vi "Save Results Time Steps.vi"() -> (5 "Plug in titles":string[](array[string]), 7 "Plug in values":string[](array[string]))   [LabVIEW 2020]
uses:
  <vilib>/Analysis/baseanly.llb/Mean (DBL).vi
  Globals/Meas_global.vi
  Globals/Dynamic_call_global.ph.vi
  <vilib>/Analysis/NI_AALBase.lvlib
  Controls/Post_Process.ctl
  Controls/Setup.ctl
panel:
  out "End time":dbl
  out "Start time":dbl
  in  "Subset time (s)":dbl=1.0 format="%.3f"
  out "Loop number":i32
  out "Number of Subsets":i32
  in  "Max Number of Subsets":i32=50
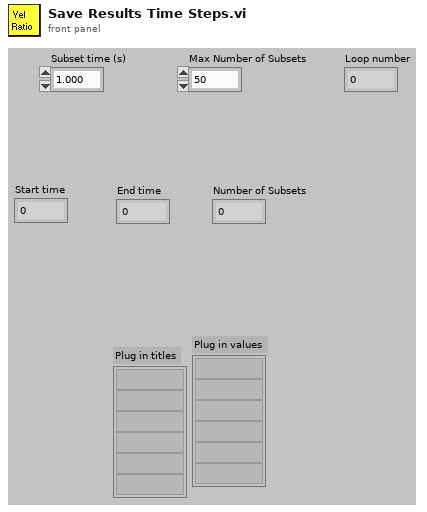
[diagram p1: front panel]
types:
  T1 = typedef "Setup.ctl" = enum16{"Run Program", "Show Setup", "Save Current Setup", "Setup Front Panel"}
  T2 = typedef "Post_Process.ctl" = enum16{"Take New Data", "Post Process Raw Data File"}
  T3 = enum16{"Save no data", "Save data in new files", "Save data in existing files"}
  T4 = typedef "Time_Trace_Cluster.ctl" = cluster{"Weighting":dbl[], "Time (s)":dbl[], "Voltage":dbl[], "Eng Values":dbl[]}
  T5 = typedef "Analysis_info_cluster.ctl" = cluster{"Colour":u32, "Inst type":T6, "Inst name":string, "Symbol":string, "Code name":string, "Extra Info":string, "Inst Array":T7, "Extra Titles":string[], "Extra Values":string[], "U":dbl, "u^2":dbl, "u^3":dbl, "u^4":dbl, "Skew_u":dbl, "Kurt_u":dbl, "Sd Error in Mean":dbl, "% u'/U":dbl, "X":dbl, "Y":dbl, "Z":dbl, "Timescale integral Estimate":dbl, "Sd Error in Variance":dbl, "Calib File":path, "Calib Constants":dbl[], "Output Position":bool, "Stats":enum16{"None", "Basic", "Full"}, "Av Sampling Rate":dbl, "Av No of Samples":dbl, "Total Meas Time (s)":dbl, "ADAM Ch Name":string, "Max value":dbl, "Min value":dbl, "Req Sample Rate Hz":dbl, "Sync Delay Time (s)":dbl, "Ch No":i16, "Device":string, "Use Latest Calib":bool, "Port":string, "Metadata Ch Names":string[], "Metadata Ch Values":string[], "Label":string}
  T6 = typedef "Inst_type.ctl" = enum16{"Raw voltage", "Raw with zero offsetting", "Propeller anemometer", "Pressure Transducer", "Pitot-static tube", "Hot wire", "Cross wire 1", "Cross wire 2", "Generic Linear", "Generic Polynomial", "Generic BackPoly", "Fast FID", "Thermocouple", "Cold wire", "Pulsed Wire", "LDA Vel", "LDA Tran time", "LDA Arr time", "Microphone"}
  T7 = typedef "Instrument_Array.ctl" = enum16{"PWA", "LDA", "Analogue"}
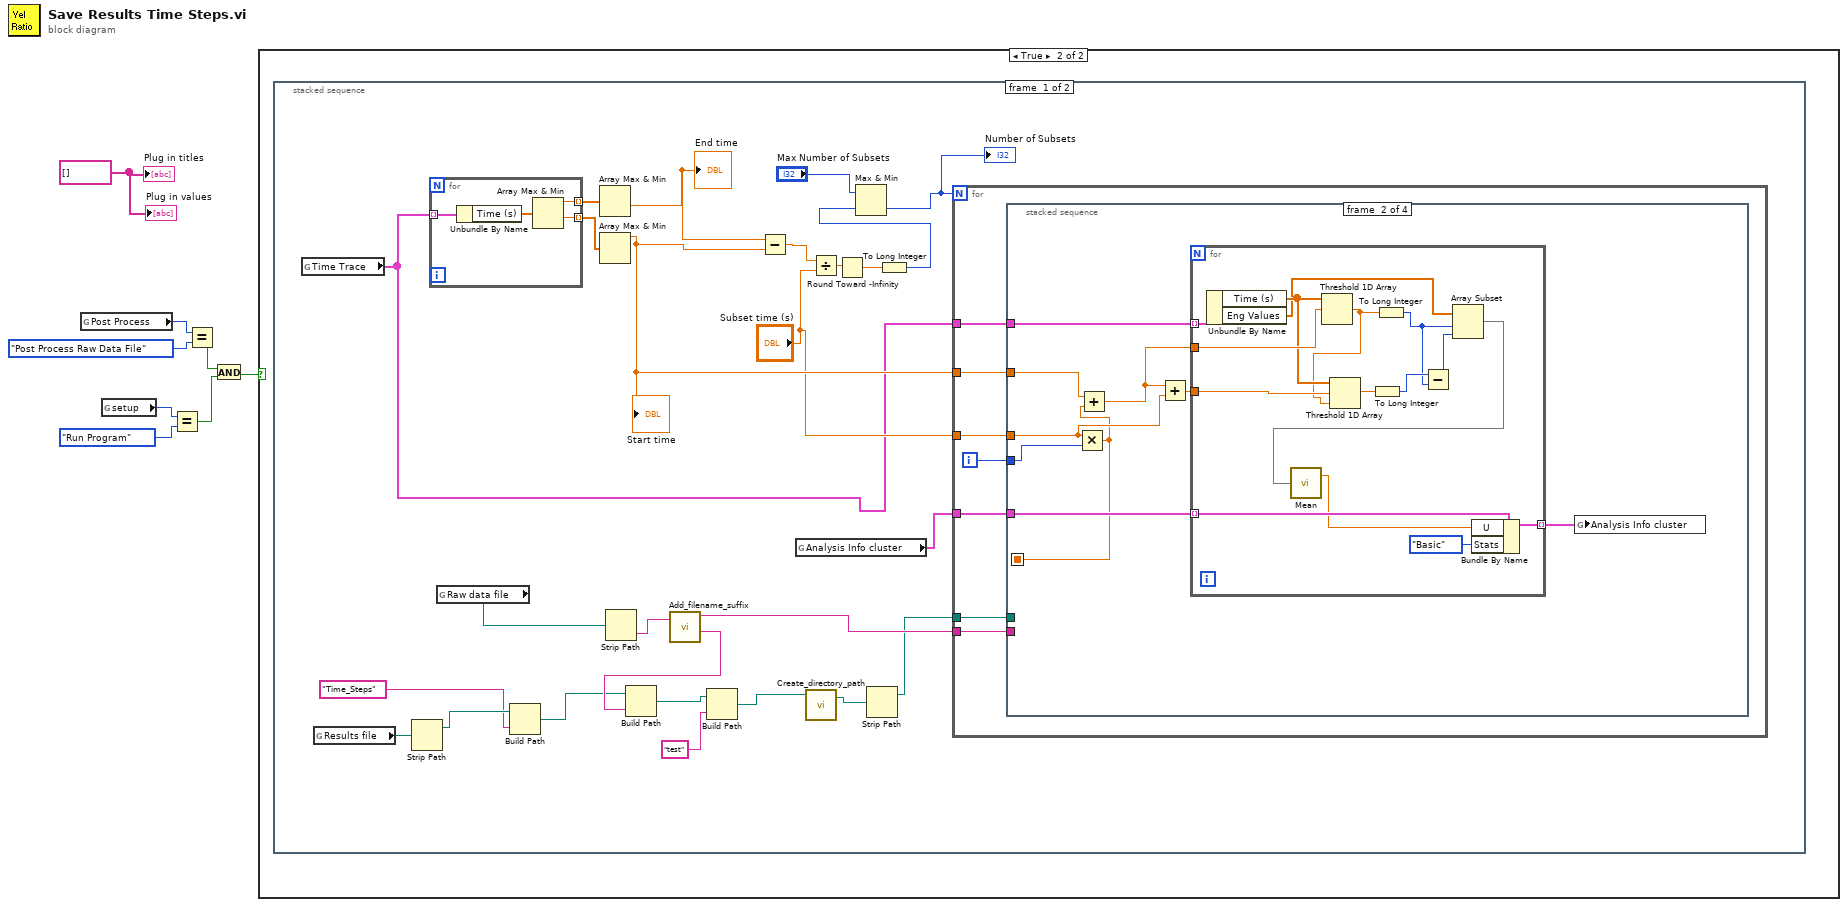
[diagram p0: block diagram]
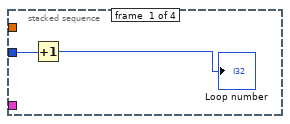
[diagram p3: hidden frame]
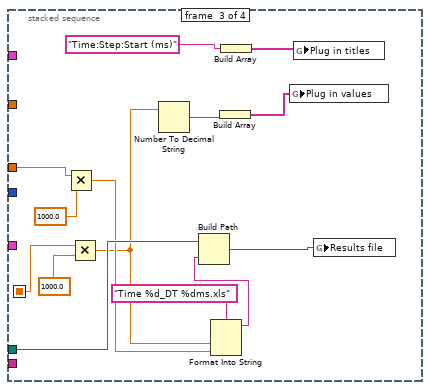
[diagram p4: hidden frame]
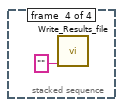
[diagram p5: hidden frame]
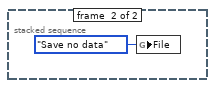
[diagram p6: hidden frame]
diagram:
  w8 = string[] [] ("Plug in titles")
  n1 = global read "Meas_global.vi" "Post Process"() -> (w6:T2)
  n2 = global read "Meas_global.vi" "setup"() -> (w4:T1)
  n3 = Equal?(x=w4, y=Setup."Run Program" ("setup")) -> (x = y?=w1:bool)
  n4 = Equal?(x=w6, y=Post_Process."Post Process Raw Data File" ("Post Process")) -> (x = y?=w3:bool)
  n5 = And(x=w3, y=w1) -> (x .and. y?=w2:bool)
  n6 = case shown="True" w2 {
    frame False {
    }
    frame True {
      n7 = stacked-sequence {
        frame #0 {
          n8 = global read "Meas_global.vi" "Time Trace"() -> (w14:T4[])
          n9 = global read "Meas_global.vi" "Results file"() -> (w13:path)
          n10 = Strip Path(path=w13) -> (stripped path=w12:path)  [unwired: 1 out]
          n11 = for {
            tunnel: w14 -> [w86] mode=indexing
            tunnel: [w84] -> w15 mode=indexing
            tunnel: [w83] -> w16 mode=indexing
            n12 = Unbundle By Name(w86) -> ("Time (s)"=w85:dbl[])
            n13 = Array Max & Min(array=w85) -> (max value=w84:dbl, min value=w83:dbl)  [unwired: 2 out]
          }
          n14 = global read "Meas_global.vi" "Raw data file"() -> (w23:path)
          n15 = Build Path(base path=w12, name or relative path="Time_Steps") -> (appended path=w10:path)
          n16 = Array Max & Min(array=w15) -> (min value=w17:dbl)  [unwired: 3 out]
          "End time" <- w17
          n17 = Array Max & Min(array=w16) -> (max value=w21:dbl)  [unwired: 3 out]
          "Start time" <- w21
          n18 = Strip Path(path=w23) -> (name=w24:string)  [unwired: 1 out]
          n19 = call "Add_filename_suffix.vi"("Filename"=w24) -> ("Original Suffix"=w30:string, "Base name"=w31:string)  [unwired: 1 in, 2 out]
          n20 = Build Path(base path=w10, name or relative path=w31) -> (appended path=w25:path)
          n21 = Build Path(base path=w25, name or relative path="test") -> (appended path=w27:path)
          n22 = Subtract(x=w17, y=w21) -> (x-y=w18:dbl)
          n23 = global read "Meas_global.vi" "Analysis Info cluster"() -> (w22:T5[])
          n24 = call "Create_directory_path.vi"("Path name"=w27) -> ("Path name Out"=w28:path)  [unwired: 2 in, 1 out]
          n25 = Divide(x=w18, y="Subset time (s)") -> (x/y=w19:dbl)
          n26 = Round Toward -Infinity(1:w19) -> (0:w33:dbl)
          n27 = Strip Path(path=w28) -> (stripped path=w29:path)  [unwired: 1 out]
          n28 = To Long Integer(number=w33) -> (32bit integer=w34:i32)
          n29 = Max & Min(x="Max Number of Subsets", y=w34) -> (min(x,y)=w9:i32)  [unwired: 1 out]
          "Number of Subsets" <- w9
          n30 = for {
            N: w9 -> [_]
            tunnel: "Subset time (s)" -> [w39]
            tunnel: w21 -> [w41]
            tunnel: w14 -> [w40]
            tunnel: w22 -> [w38]
            tunnel: w30 -> [w37]
            tunnel: w29 -> [w36]
            i -> [w35]
            n31 = stacked-sequence {
              seq-local: [_ w44 _ _] -> [_ _ w78 _]
              tunnel: w41 -> [_ w52 _ _]
              tunnel: w40 -> [_ w51 _ _]
              tunnel: w39 -> [_ w50 w75 _]
              tunnel: w38 -> [_ w48 _ _]
              tunnel: w37 -> [_ _ _ _]
              tunnel: w36 -> [_ _ w81 _]
              tunnel: w35 -> [w43 w46 _ _]
              frame #0 {
                n32 = Increment(x=w43) -> (x+1=→"Loop number":i32)
              }
              frame #1 {
                n33 = Multiply(x=w50, y=w46) -> (x*y=w44:dbl)
                n34 = Add(x=w52, y=w44) -> (x+y=w45:dbl)
                n35 = Add(x=w45, y=w50) -> (x+y=w49:dbl)
                n36 = for {
                  tunnel: w51 -> [w67] mode=indexing
                  tunnel: w45 -> [w66]
                  tunnel: w49 -> [w64]
                  tunnel: w48 -> [w56] mode=indexing
                  tunnel: [w54] -> w47 mode=indexing
                  n37 = Unbundle By Name(w67) -> ("Time (s)"=w65:dbl[], "Eng Values"=w61:dbl[])
                  n38 = Threshold 1D Array(2:w66, 3:w65) -> (0:w62:dbl)  [unwired: 1 in]
                  n39 = Threshold 1D Array(1:w62, 2:w64, 3:w65) -> (0:w63:dbl)
                  n40 = To Long Integer(number=w63) -> (32bit integer=w60:i32)
                  n41 = To Long Integer(number=w62) -> (32bit integer=w59:i32)
                  n42 = Subtract(x=w60, y=w59) -> (x-y=w58:i32)
                  n43 = Array Subset(array=w61, index=w59, length=w58) -> (w57:dbl[])
                  n44 = call-poly <vilib>:"Mean.vi"("X"=w57) -> ("mean"=w55:dbl)  [unwired: 1 out]
                  n45 = Bundle By Name(cluster=w56, "U"=w55, "Stats"=enum16{"None", "Basic", "Full"}."Basic") -> (w54:T5)
                }
                n46 = global write "Meas_global.vi" "Analysis Info cluster"(w47) -> ()
              }
              frame #2 {
                n47 = Multiply(x=w75, y=1000.0) -> (x*y=w73:dbl)
                n48 = Multiply(x=w78, y=1000.0) -> (x*y=w68:dbl)
                n49 = Number To Decimal String(number=w68) -> (decimal integer string=w69:string)  [unwired: 1 in]
                n50 = Format Into String(format string="Time %d_DT %dms.xls", w68, w73) -> (resulting string=w80:string)  [unwired: 2 in, 1 out]
                n51 = Build Path(base path=w81, name or relative path=w80) -> (appended path=w79:path)
                n52 = Build Array(w69) -> (w70:string[])
                n53 = Build Array("Time:Step:Start (ms)") -> (w72:string[])
                n54 = global write "Dynamic_call_global.ph.vi" "Plug in values"(w70) -> ()
                n55 = global write "Dynamic_call_global.ph.vi" "Plug in titles"(w72) -> ()
                n56 = global write "Meas_global.vi" "Results file"(w79) -> ()
              }
              frame #3 {
                n57 = call "Write_Results_file.vi"("Setup filename"="") -> ()  [unwired: 2 in, 4 out]
              }
            }
          }
        }
        frame #1 {
          n58 = global write "Meas_global.vi" "File"(T3."Save no data" ("File")) -> ()
        }
      }
    }
  }
  "Plug in values" <- w8
  "Plug in titles" <- w8
